vi "00-StartVI-Status.vi"(8 "error in (no error)":errorcluster caption="错误输入（无错误）", 10 "DataIn":cluster{"Data":string, "Status":bool}, 11 "Step":enum16{"Initial", "Write", "Read"}(ring)) -> (0 "error out":errorcluster caption="错误输出", 3 "DataOut":cluster{"Data":string, "Status":bool})   [LabVIEW 2017]
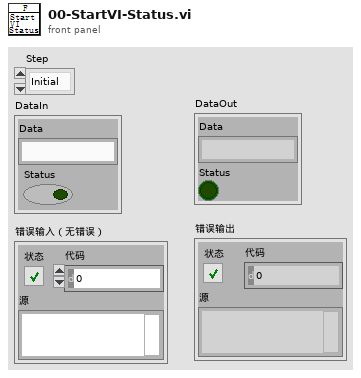
[diagram p1: front panel]
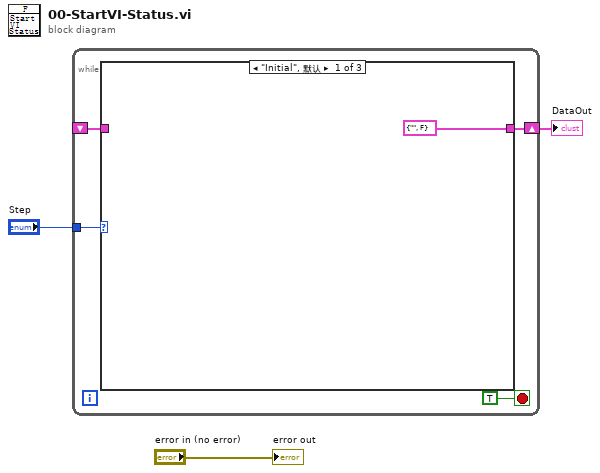
[diagram p0: block diagram]
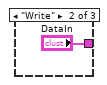
[diagram p2: hidden frame]
diagram:
  n1 = while {
    tunnel: "Step" -> [w7]
    shift-right: [w5] -> w2
    shift-left: _ -> [w4]
    stop <- TRUE stop-if-true
    n2 = case shown="\"Initial\", 默认" w7 {
      tunnel: [cluster{"Data":string, "Status":bool} {"Data"="", "Status"=FALSE} "DataIn" w10] -> w5
      tunnel: w4 -> [_ _ w10]
      frame "Initial", Default {
      }
      frame "Write" {
      }
      frame "Read" {
      }
    }
  }
  "DataOut" <- w2
  "error out" <- "error in (no error)"
